vi "Global_SM Write_Data Out.vi"() -> ()   [LabVIEW 2016, in "TemplateActuator.lvlib"]
uses:
  TemplateActuator.lvlib
panel:
  in  "TemplateActuator_SM_Int":i32
  in  "TemplateActuator_SM_Bool":bool
  in  "TemplateActuator_SM_DBL":dbl
  # "The Names of the Data items in the Global Variable MUST describe who the Single Writer is\nNaming Convention of all Data Items is:   \nLib Name_Loop Name (SM or SEN or ACT)_Data Name\nExamples:\nDrive_ACT_X axis\nGameController_SEN_JoystickLeft\nHopper_SM_AgitatorSpeed"
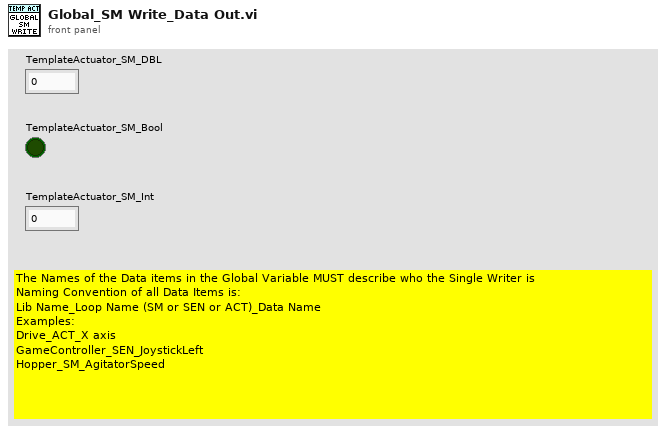
[diagram p1: front panel]
diagram:
